vi "New JSON ({Boolean}).vi"(7 "key":string, 8 "error in (no error)":errorcluster, 10 "value":bool) -> (0 "error out":errorcluster, 3 "JSON Value out":refnum<class "JSON Value.lvclass">)   [LabVIEW 2017, in "JSON Value.lvclass"]
doc: "Create a new JSON Object initialized with the given key value pair."
uses:
  JSON Value.lvclass
  Object/Insert Value/Insert Value (Boolean).vi
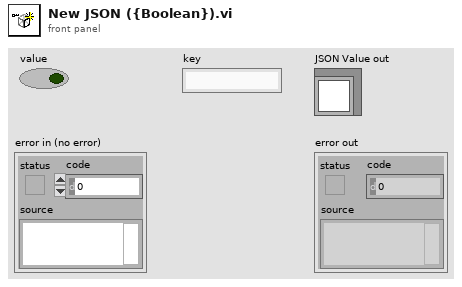
[diagram p1: front panel]
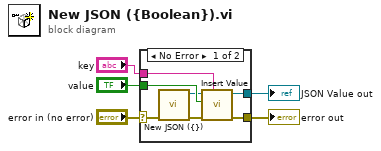
[diagram p0: block diagram]
diagram:
  n1 = case shown="No Error" "error in (no error)" {
    selector: "error in (no error)" -> [w12 w13]
    tunnel: [w11 w13] -> w4
    tunnel: [w10 _] -> w3
    tunnel: "key" -> [w9 _]
    tunnel: "value" -> [w8 _]
    frame No Error {
      n2 = call "New JSON ({}).vi"("error in (no error)"=w12) -> ("error out"=w7:errorcluster, "JSON Value out"=w6:refnum<class "JSON Value.lvclass">)  [unwired: 9 in]
      n3 = call-poly "Insert Value.vi"("key"=w9, "error in (no error)"=w7, "value"=w8, "JSON Value in"=w6) -> ("error out"=w11:errorcluster, "JSON Value out"=w10:refnum<class "JSON Value.lvclass">)  [unwired: 5 in, 1 out]
    }
    frame Error {
    }
  }
  "error out" <- w4
  "JSON Value out" <- w3
